vi "DrawOverlay.vi"(8 "error in (no error)":errorcluster, 11 "menu in":refnum<class "menu.lvclass">) -> (0 "error out":errorcluster, 3 "menu out":refnum<class "menu.lvclass">)   [LabVIEW 2009, in "menu.lvclass"]
uses:
  menu.lvclass
  menu.lvclass/menu.ctl
  Overlay/overlay.lvclass
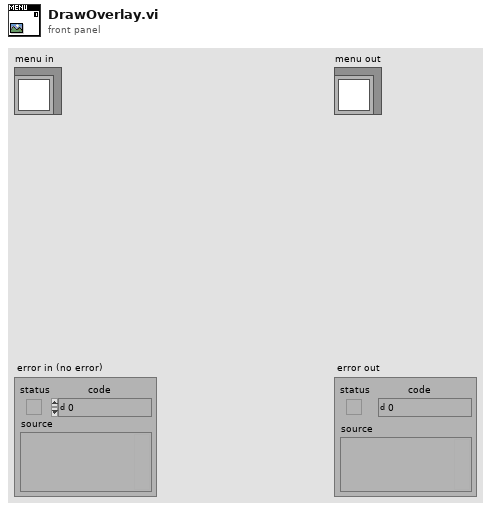
[diagram p1: front panel]
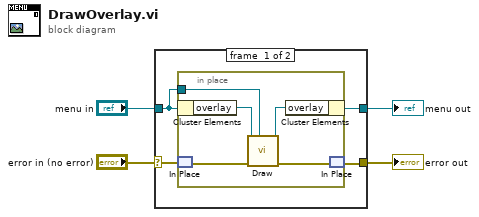
[diagram p0: block diagram]
diagram:
  n1 = case shown="No Error" "error in (no error)" {
    selector: "error in (no error)" -> [w7 w15]
    tunnel: [w6 w15] -> w1
    tunnel: [w8 w14] -> w3
    tunnel: "menu in" -> [w5 w14]
    frame #0 {
      n2 = in-place {
        in-place-border: w5 -> [w9]
        n3 = in-place-cluster #1(w5) -> ("overlay"=w11:refnum<class "overlay.lvclass">)
        n4 = in-place-match #2(w7) -> (w13:errorcluster)
        n5 = call "Draw.vi"("menu in"=w9, "error in (no error)"=w13, "overlay in"=w11) -> ("error out"=w12:errorcluster, "overlay out"=w10:refnum<class "overlay.lvclass">)  [unwired: 7 in]
        n6 = in-place-cluster #1("overlay"=w10) -> (w8:refnum<class "menu.lvclass">)
        n7 = in-place-match #2(w12) -> (w6:errorcluster)
      }
    }
    frame #1 {
    }
  }
  "menu out" <- w3
  "error out" <- w1
